vi "Derivative.vi"   [LabVIEW 2020, in "NI_AdvCtrl_continuous linear.lvlib"]
doc: "LabVIEW no longer supports this VI. You can obtain similar functionality by installing the LabVIEW Simulation Module.\n\nCalculates the derivative of a continuous signal, where the formula output(n)=(input(n)-input(n-1))/dt is used. This element is a specific transfer function with H(s)=s."
uses:
  <vilib>/addons/control/advanced/NI_AdvCtrl_continuous linear.lvlib
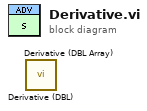
[diagram p0: block diagram]
diagram:
  n1 = call <vilib>:"Derivative (DBL).vi"() -> ()  [unwired: 5 in, 1 out]
  n2 = call <vilib>:"Derivative (DBL Array).vi"() -> ()  [unwired: 5 in, 1 out]
